vi "Conv_JSON_6 (SubVI).vi"(9 "data":cluster{"name":string, "value":T1}={"name"="i_range", "value"=enum."auto"}, 11 "Cluster":T2) -> (3 "String":string)   [LabVIEW 2015]
uses:
  Ctrl/I_range.ctl
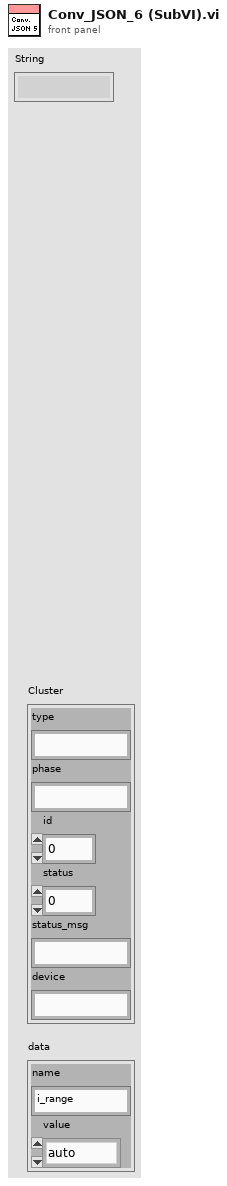
[diagram p1: front panel]
types:
  T1 = typedef "I_range.ctl" = enum16{"off", "18 µA", "180 µA", "1.8 mA", "18 mA", "180 mA", "2 A", "10 A", "auto"}
  T2 = cluster{"type":string, "phase":string, "id":u8, "status":i32, "status_msg":string, "device":string}
  T3 = cluster{"type":string, "phase":string, "id":u8, "status":i32, "status_msg":string, "device":string, "data":cluster{"name":string, "value":string}}
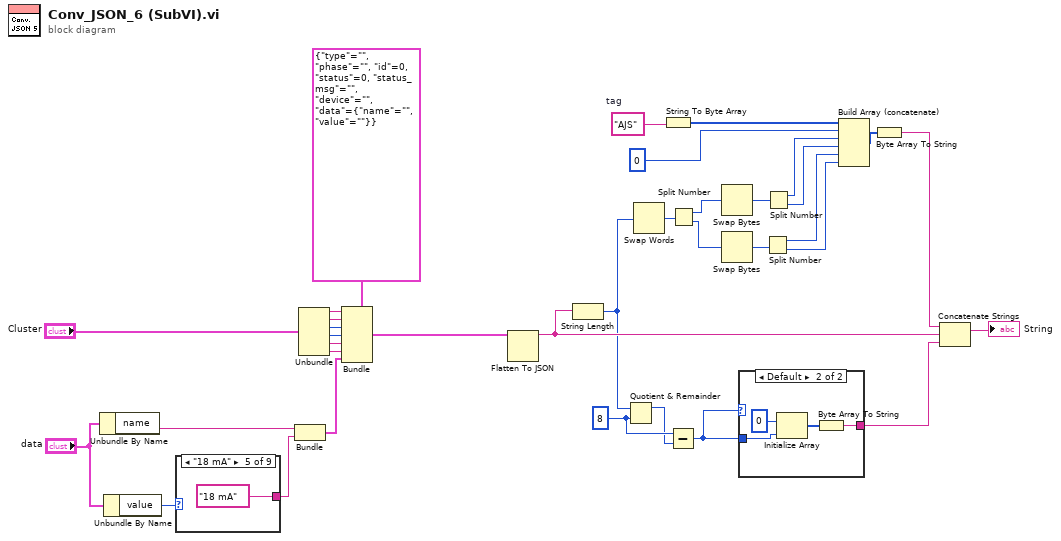
[diagram p0: block diagram]
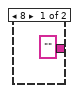
[diagram p2: hidden frame]
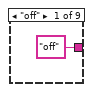
[diagram p3: hidden frame]
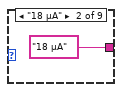
[diagram p4: hidden frame]
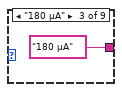
[diagram p5: hidden frame]
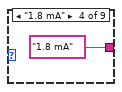
[diagram p6: hidden frame]
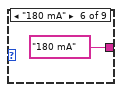
[diagram p7: hidden frame]
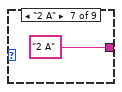
[diagram p8: hidden frame]
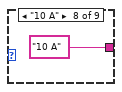
[diagram p9: hidden frame]
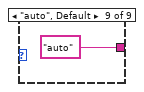
[diagram p10: hidden frame]
diagram:
  w5 = 8 ("y")
  w30 = "AJS"  # tag
  n1 = Unbundle By Name("data") -> ("name"=w8:string)
  n2 = Unbundle By Name("data") -> ("value"=w12:T1)
  n3 = case shown="\"18 mA\"" w12 {
    tunnel: ["off" ("type") "18 µA" ("type") "180 µA" ("type") "1.8 mA" ("type") "18 mA" ("type") "180 mA" ("type") "2 A" ("type") "10 A" ("type") "auto" ("type")] -> w7
    frame "off" {
    }
    frame "18 µA" {
    }
    frame "180 µA" {
    }
    frame "1.8 mA" {
    }
    frame "18 mA" {
    }
    frame "180 mA" {
    }
    frame "2 A" {
    }
    frame "10 A" {
    }
    frame "auto", Default {
    }
  }
  n4 = Bundle("name"=w8, "type"=w7) -> (w6:cluster{"name":string, "type":string})  [unwired: 1 in]
  n5 = Unbundle("Cluster") -> ("type"=w19:string, "phase"=w18:string, "id"=w17:u8, "status"=w16:i32, "status_msg"=w15:string, "device"=w14:string)
  n6 = Bundle(cluster=T3 {"type"="", "phase"="", "id"=0, "status"=0, "status_msg"="", "device"="", "data"={"name"="", "value"=""}}, "type"=w19, "phase"=w18, "id"=w17, "status"=w16, "status_msg"=w15, "device"=w14, "data"=w6) -> (w11:T3)
  n7 = Flatten To JSON(anything=w11) -> (JSON string=w34:string)  [unwired: 2 in, 1 out]
  n8 = String Length(string=w34) -> (length=w2:i32)
  n9 = Quotient & Remainder(x=w2, y=w5) -> (x-y*floor(x/y)=w4:i32)  [unwired: 1 out]
  n10 = Swap Words(1:w2) -> (0:w33:i32)
  n11 = String To Byte Array(string=w30) -> (unsigned byte array=w29:u8[])
  n12 = Subtract(x=w5, y=w4) -> (x-y=w3:i32)
  n13 = Split Number(x=w33) -> (hi(x)=w32:u16, lo(x)=w31:u16)
  n14 = Swap Bytes(anything=w32) -> (byte swapped=w24:u16)
  n15 = Swap Bytes(anything=w31) -> (byte swapped=w25:u16)
  n16 = case shown="Default" w3 {
    tunnel: ["" ("string") w47] -> w1
    tunnel: w3 -> [_ w46]
    frame 8 {
    }
    frame Default {
      n17 = Initialize Array(u8 0 ("element"), w46) -> (w48:u8[])
      n18 = Byte Array To String(unsigned byte array=w48) -> (string=w47:string)
    }
  }
  n19 = Split Number(x=w25) -> (hi(x)=w21:u8, lo(x)=w20:u8)
  n20 = Split Number(x=w24) -> (hi(x)=w23:u8, lo(x)=w22:u8)
  n21 = Build Array (concatenate)(w29, u8 0, w23, w22, w21, w20) -> (w27:u8[])
  n22 = Byte Array To String(unsigned byte array=w27) -> (string=w26:string)
  n23 = Concatenate Strings(w26, w34, w1) -> (→"String":string)
